vi "SetRowHeaderFont.vi"(0 "reference in":refnum<class "DataGridView.lvclass">, 5 "FontName":string, 7 "emSize":sgl, 9 "style":i32(ring) items=["Regular"=0, "Bold"=1, "Italic"=2, "Underline"=4, "Strikeout"=8], 11 "error in (no error)":errorcluster) -> (4 "reference out":refnum<class "DataGridView.lvclass">, 15 "error out":errorcluster)   [LabVIEW 2018, in "DataGridView.lvclass"]
doc: "Sets the font and size for the the Column Headers. \n\nIf the font family cannot be found it will resolve to the default font"
uses:
  DataGridView.lvclass
  System.Windows.Forms
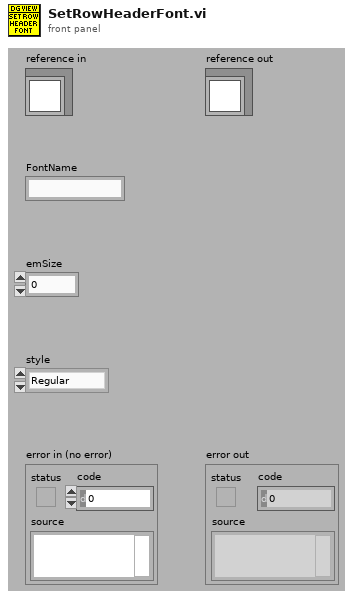
[diagram p1: front panel]
types:
  T1 = typedef "DataGridView.lvclass/ObjectAttributes.ctl" = cluster{"DataGridView":refnum<k24>, "SelectionChangedEvent":refnum<user-event>, "SelectionChanged callback ref":refnum<k27>, "LastSelectedRowIndex":i32}
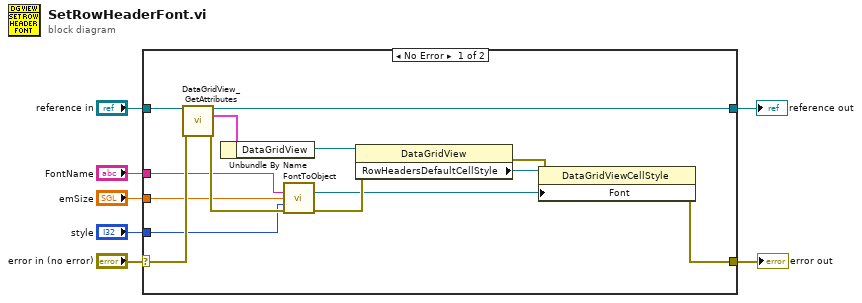
[diagram p0: block diagram]
diagram:
  n1 = case shown="No Error" "error in (no error)" {
    selector: "error in (no error)" -> [w21 w23]
    tunnel: [w14 w23] -> w6
    tunnel: [w18 w22] -> w4
    tunnel: "reference in" -> [w19 w22]
    tunnel: "FontName" -> [w10 _]
    tunnel: "emSize" -> [w9 _]
    tunnel: "style" -> [w8 _]
    frame No Error {
      n2 = call "DataGridView_GetAttributes.vi"("reference in"=w19, "error in (no error)"=w21) -> ("reference out"=w18:refnum<class "DataGridView.lvclass">, "Data"=w20:T1, "error out"=w13:errorcluster)  [unwired: 10 in, 1 out]
      n3 = Unbundle By Name(w20) -> ("DataGridView"=w17:refnum<k24>)
      n4 = call "FontToObject.vi"("FontName"=w10, "emSize"=w9, "style"=w8, "error in (no error)"=w13) -> ("FontObject"=w11:refnum<k24>, "error out"=w12:errorcluster)  [unwired: 10 in]
      n5 = property class="DataGridView"(reference=w17, error in=w12) -> (error out=w15:errorcluster, "RowHeadersDefaultCellStyle"=w16:refnum<k24>)  [unwired: 1 out]
      n6 = property class="DataGridViewCellStyle"(reference=w16, error in=w15, "Font"=w11) -> (error out=w14:errorcluster)  [unwired: 1 out]
    }
    frame Error {
    }
  }
  "error out" <- w6
  "reference out" <- w4
